vi "pid.calculate_trapezoidal.vi"(6 "sampling_time (s)":dbl, 9 "Td":dbl, 10 "Ti":dbl, 11 "Kc":dbl) -> (2 "a1...an":dbl[](array[numeric]), 3 "b0...bn":dbl[](array[numeric]))   [LabVIEW 2015, in "discrete_control_systems.lvlib"]
doc: "Calculates the gains for a discrete difference equation from the PID controller parameters using the trapezoidal discretization method.\n\nThe implemented controller has the following equation in the LaPlace domain, where U(s) is the controller output:\n\nU(s) = Kc * ( 1 + 1/(Ti*s) + Td*s )"
uses:
  discrete_control_systems.lvlib
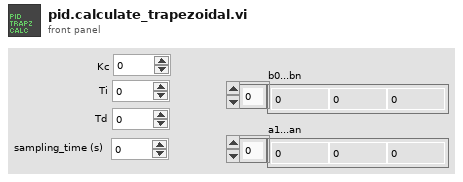
[diagram p1: front panel]
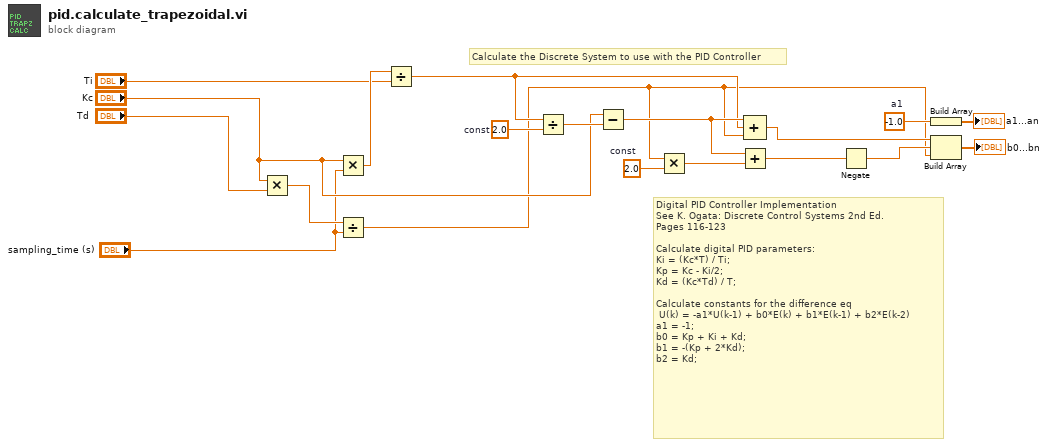
[diagram p0: block diagram]
diagram:
  w17 = -1.0  # a1
  w14 = 2.0  # const
  w10 = 2.0  # const
  # "Digital PID Controller Implementation\nSee K. Ogata: Discrete Control Systems 2nd Ed.\nPages 116-123\n\nCalculate digital PID parameters:\nKi = (Kc*T) / Ti;\nKp = Kc - Ki/2;\nKd = (Kc*Td) / T;\n\nCalculate constants for the difference eq\n U(k) = -a1*U(k-1) + b0*E(k) + b1*E(k-1) + b2*E(k-2)\na1 = -1;\nb0 = Kp + Ki + Kd;\nb1 = -(Kp + 2*Kd);\nb2 = Kd;"
  # "Calculate the Discrete System to use with the PID Controller"
  n1 = Multiply(x="Kc", y="Td") -> (x*y=w11:dbl)
  n2 = Multiply(x="Kc", y="sampling_time (s)") -> (x*y=w8:dbl)
  n3 = Divide(x=w11, y="sampling_time (s)") -> (x/y=w4:dbl)
  n4 = Divide(x=w8, y="Ti") -> (x/y=w12:dbl)
  n5 = Divide(x=w12, y=w10) -> (x/y=w9:dbl)
  n6 = Subtract(x="Kc", y=w9) -> (x-y=w13:dbl)
  n7 = Multiply(x=w4, y=w14) -> (x*y=w15:dbl)
  n8 = Add(x=w13, y=w15) -> (x+y=w16:dbl)
  n9 = Compound Arithmetic op=ADD(w13, w12, w4) -> (w18:dbl)
  n10 = Negate(x=w16) -> (-x=w19:dbl)
  n11 = Build Array(w17) -> (→"a1...an":dbl[])
  n12 = Build Array(w18, w19, w4) -> (→"b0...bn":dbl[])
